vi "Tenerowicz_Target_C_2.vi"   [LabVIEW 2023]
uses:
  <vilib>/Platform/TimedLoop/XDataNode/timing_clust.ctl
  <vilib>/Platform/TimedLoop/XDataNode/nitl_modes.ctl
  <vilib>/Platform/TimedLoop/XDataNode/wakeup.ctl
  <vilib>/platform/TimedLoop/XDataNode/XDataNode.xnode
  <vilib>/Platform/TimedLoop/XDataNode/XDNodeRunTimeDep.lvlib
types:
  T1 = typedef "XDNodeRunTimeDep.lvlib/timing_clust.ctl" = cluster{"Expected End [f-1]":u64, "Actual End [f-1]":u64, "Finished Late? [f-1]":bool, "Expected End [i-1]":u64, "Actual End [i-1]":u64, "Finished Late? [i-1]":bool, "Expected Start [i]":u64, "Actual Start [i]":u64, "Expected Start [f]":u64, "Actual Start [f]":u64, "Source Name":string, "Structure Name":string, "Period":i64, "Deadline":i64, "Offset":i64, "Start":i64, "Priority":i32, "Timeout":i32, "Mode":T2, "Wakeup Reason":T3, "Error":errorcluster, "Source Type":string, "Secondary Source Type":string, "Global End Time":u64, "Global Start Time":u64, "Frame Duration":u64, "Iteration Duration":u64, "Assigned CPU":i32, "I/O Scan Engine Mode":u32}
  T2 = typedef "XDNodeRunTimeDep.lvlib/nitl_modes.ctl" = enum32{"No Change", "Process missed periods, maintain original phase", "Discard missed periods, maintain original phase", "Process missed periods, ignore original phase", "Discard missed periods, ignore original phase"}
  T3 = typedef "XDNodeRunTimeDep.lvlib/wakeup.ctl" = enum32{"Normal", "Aborted", "Asynchronous wakeup", "Timing source error", "Timed loop error", "Timeout"}
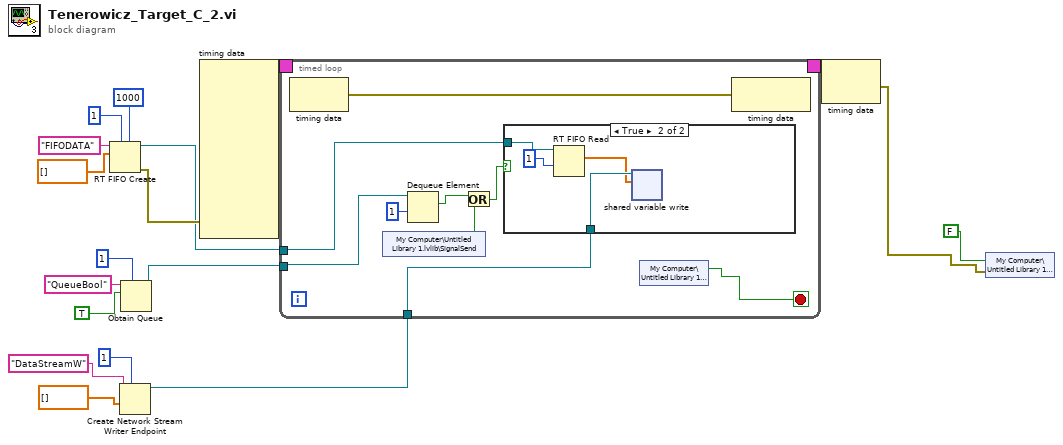
[diagram p0: block diagram]
diagram:
  n1 = RT FIFO Create(0:"FIFODATA" ("name (unnamed)"), 1:dbl[] [] ("type"), 4:u32 1 ("size (10)"), 6:u32 1000 ("elements in array (1)")) -> (8:w5:refnum<k33>, 11:w6:errorcluster)  [unwired: 4 in, 1 out]
  n2 = Create Network Stream Writer Endpoint(7:1 ("writer buffer size"), 9:dbl[] [] ("type"), 11:"DataStreamW" ("writer name")) -> (3:w3:refnum<k21>)  [unwired: 4 in, 1 out]
  n3 = Obtain Queue(max queue size (-1, unlimited)=1, name (unnamed)="QueueBool", element data type=TRUE) -> (queue out=w4:refnum<queue>)  [unwired: 2 in, 2 out]
  n4 = node-c288(w6) -> (w18:T1)  [unwired: 9 in]
  n5 = timed-loop {
    timing: w18 -> [_]
    timing-out: [_] -> w17
    tunnel: w5 -> [w23]
    tunnel: w4 -> [w26]
    tunnel: w3 -> [w24]
    stop <- w19 stop-if-true
    n6 = node-c288() -> (w27:errorcluster)  [unwired: 1 in]
    n7 = shared-variable "My Computer\\Untitled Library 1.lvlib\\SignalSend"() -> (w20:bool)  [unwired: 1 in, 1 out]
    n8 = Dequeue Element(queue=w26, timeout in ms (-1)=1) -> (element=w22:bool)  [unwired: 1 in, 3 out]
    n9 = Or(x=w22, y=w20) -> (x .or. y?=w21:bool)
    n10 = case shown="True" w21 {
      tunnel: w24 -> [_ w31]
      tunnel: w23 -> [_ w30]
      frame False {
      }
      frame True {
        n11 = RT FIFO Read(0:w30, 2:1 ("timeout in ms (0)")) -> (9:w28:dbl[])  [unwired: 2 in, 4 out]
        n12 = shared-variable-write(w31, w28) -> ()  [unwired: 2 in, 3 out]
      }
    }
    n13 = shared-variable "My Computer\\Untitled Library 1.lvlib\\Stop"() -> (w19:bool)  [unwired: 1 in, 1 out]
    n14 = node-c288(w27) -> ()  [unwired: 1 out]
  }
  n15 = node-c288(w17) -> (w2:errorcluster)
  n16 = shared-variable "My Computer\\Untitled Library 1.lvlib\\Stop"(FALSE ("Stop"), error in=w2) -> ()  [unwired: 1 out]
